vi "Process.vi"(11 "Main Controller":refnum<class "Main Controller Actor.lvclass">) -> ()   [LabVIEW 2021, in "Main Controller Actor.lvclass"]
uses:
  Main Controller Actor.lvclass
  C:/dev/LabVIEW/LabMelee/Source/Re-use Libraries/Minimal Actor Framework/Actors/Base Actor/Actor/Actor.lvclass
  Re-use Libraries/Minimal Actor Framework/Actors/Base Actor/API/Actor API.lvclass
  Main Controller Actor.lvclass/Main Controller Actor.ctl
  View.ctl
  Re-use Libraries/Utility/Utility.lvlib
  Re-use Libraries/Minimal Actor Framework/Actors/Base Actor/Actor/Front Panel State.ctl
  Re-use Libraries/Minimal Actor Framework/Actors/Base Actor/Actor/Actor.lvclass
  Re-use Libraries/Minimal Actor Framework/Messaging/Message/Message.lvclass
  Error Handler/API/Error Handler Actor API.lvclass
  Windows.ctl
  Re-use Libraries/Minimal Actor Framework/Actors/Debugger/Debugger.lvclass
  API/Main Controller Actor API.lvclass
  Views/Main/Main View.lvclass
  Views/Info/Info View.lvclass
  Views/Dev/Dev View.lvclass
  Views/Process Input/Process Input View.lvclass
  Ship.ctl
  Player.ctl
  Player Ship.ctl
panel:
  in  "View":T1
  out "View Title":string
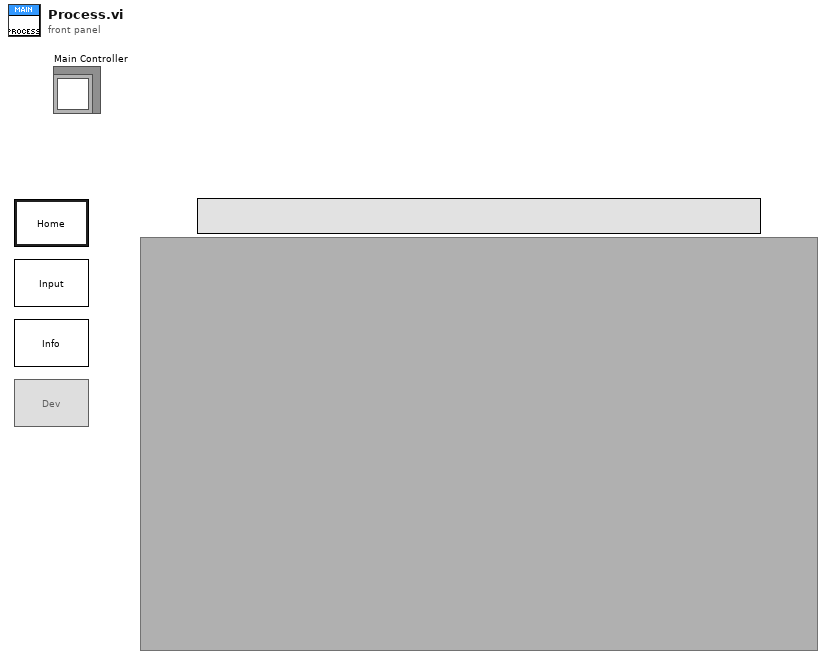
[diagram p1: front panel]
types:
  T1 = typedef "Main Controller Actor.lvclass/View.ctl" = enum32{"Main", "Boolean", "Info", "Dev"}
  T2 = typedef "Actor.lvclass/Front Panel State.ctl" = enum32{"Invalid", "Standard", "Closed", "Hidden", "Minimized", "Maximized"}
  T3 = typedef "Main Controller Actor.lvclass/Player Ship.ctl" = cluster{"Player":T4, "Ship":T5}
  T4 = typedef "Main Controller Actor.lvclass/Player.ctl" = enum16{"1", "2"}
  T5 = typedef "Main Controller Actor.lvclass/Ship.ctl" = enum16{"Arilou", "Chmmr", "Kohrah", "Slylandro"}
  T6 = typedef "Main Controller Actor.lvclass/Windows.ctl" = enum16{"Debugger"}
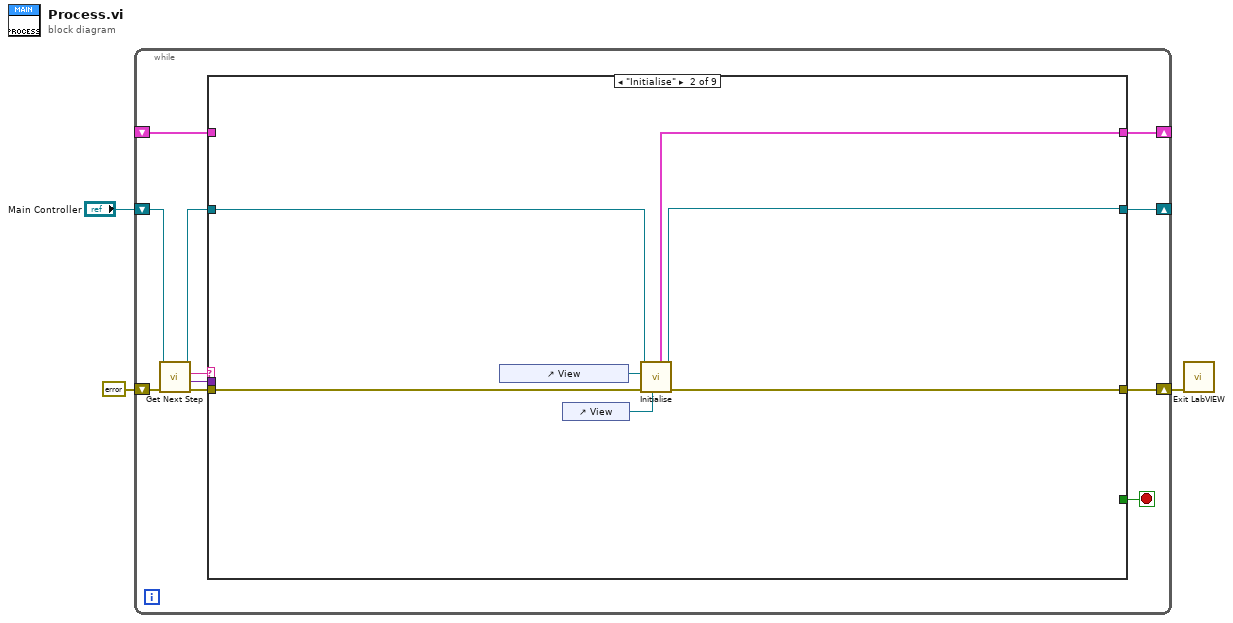
[diagram p0: block diagram]
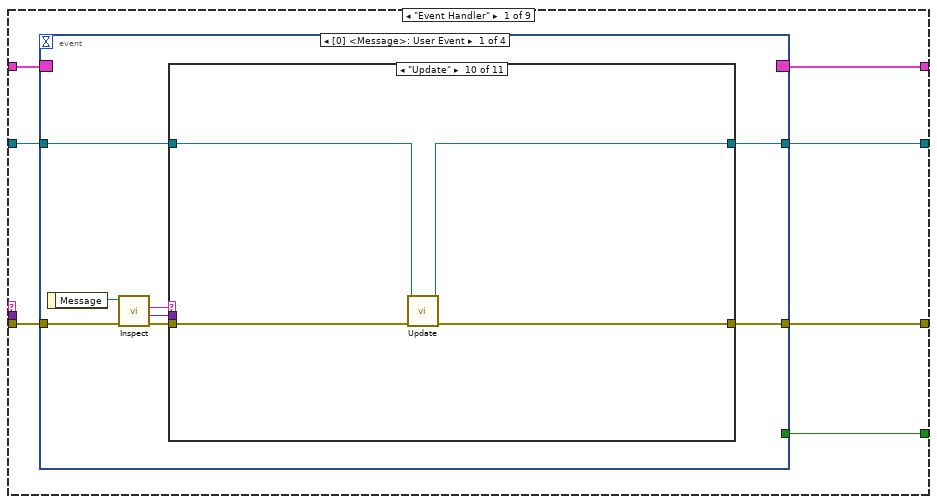
[diagram p2: hidden frame]
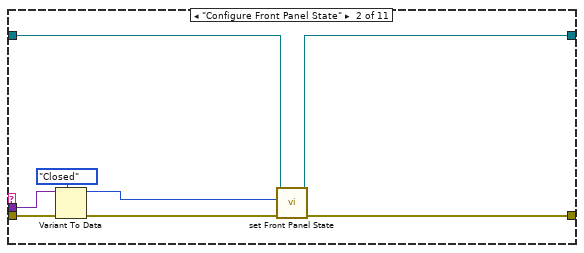
[diagram p4: hidden frame]
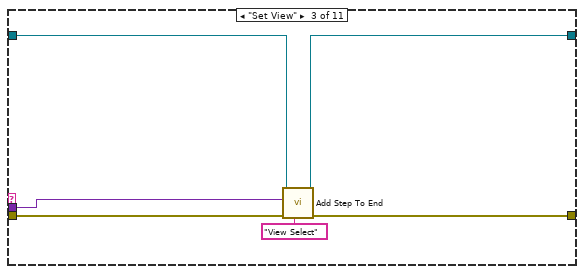
[diagram p5: hidden frame]
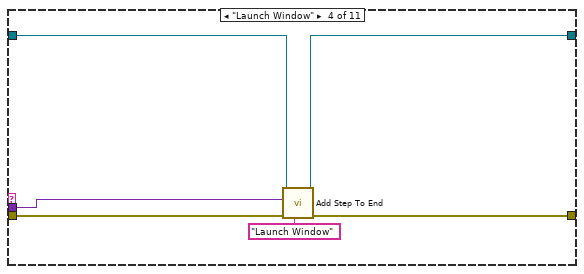
[diagram p6: hidden frame]
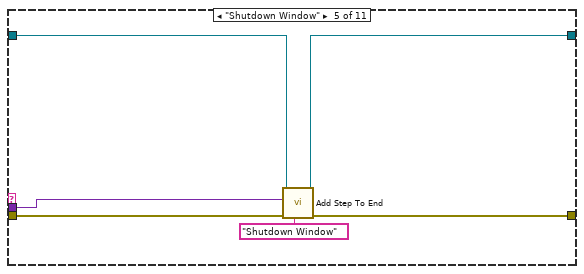
[diagram p7: hidden frame]
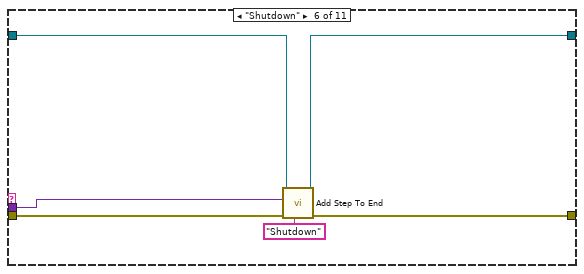
[diagram p8: hidden frame]
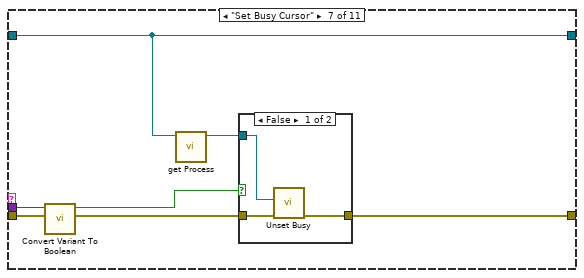
[diagram p9: hidden frame]
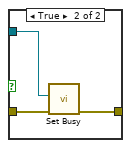
[diagram p10: hidden frame]
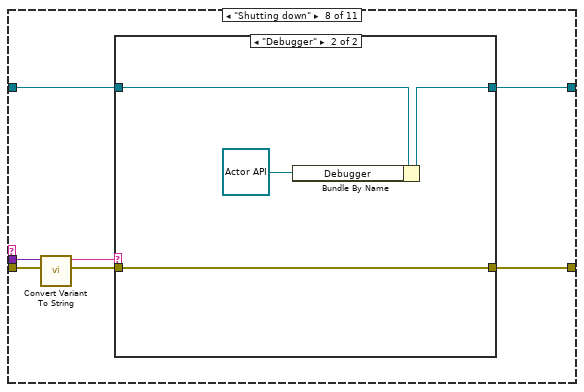
[diagram p11: hidden frame]
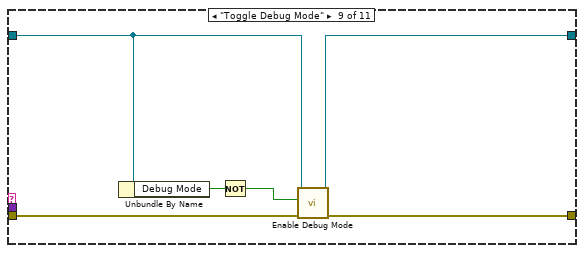
[diagram p13: hidden frame]
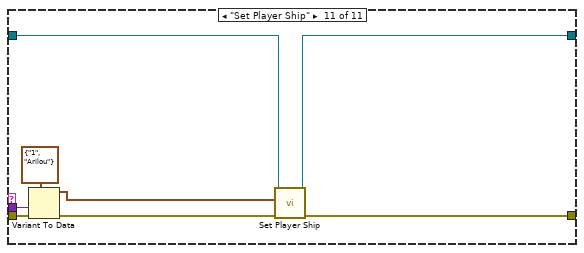
[diagram p14: hidden frame]
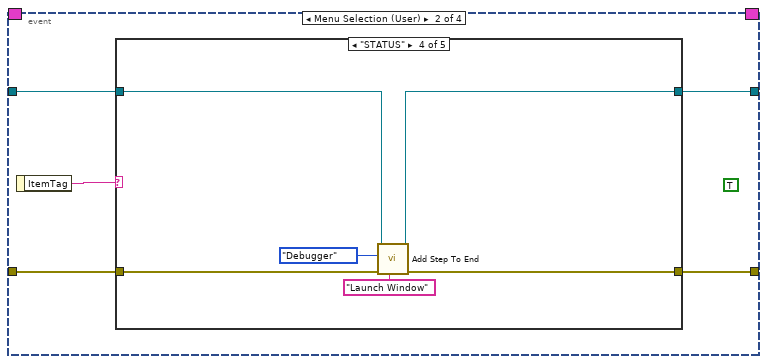
[diagram p15: hidden frame]
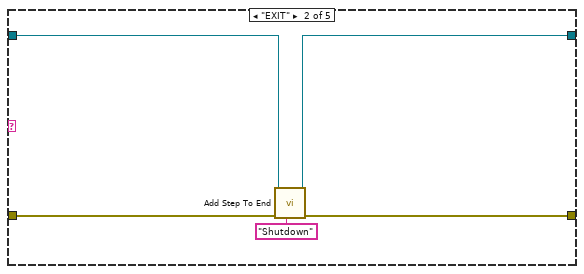
[diagram p17: hidden frame]
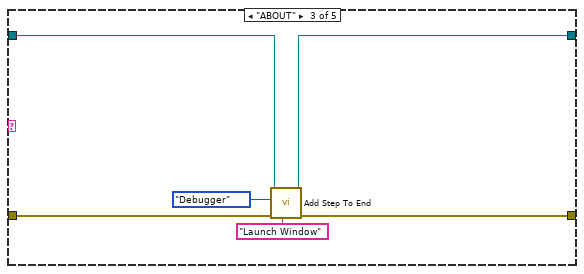
[diagram p18: hidden frame]
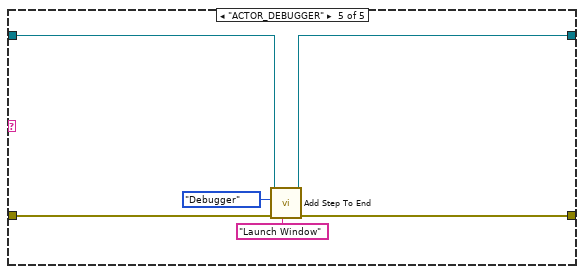
[diagram p19: hidden frame]
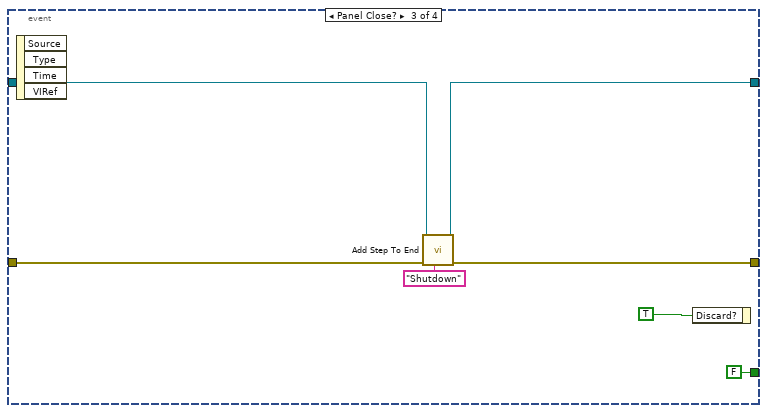
[diagram p20: hidden frame]
diagram:
  n1 = while {
    shift-right: [w9] -> _
    shift-left: "Main Controller" -> [w10]
    shift-right: [w8] -> _
    shift-left: _ -> [w7]
    shift-right: [w5] -> w2
    shift-left: errorcluster {"status"=FALSE, "code"=0, "source"=""} ("error constant") -> [w6]
    stop <- w4 stop-if-true
    n2 = call-dynamic "Get Next Step.vi"("error in (no error)"=w6, "Actor in"=w10) -> ("error out"=w12:errorcluster, "Parameter"=w11:variant, "Step"=w14:string, "Actor out"=w13:refnum<class "Main Controller Actor.lvclass">)  [unwired: 5 in, 1 out]
    n3 = case shown="\"Initialise\"" w14 {
      tunnel: w13 -> [w19 w154 w162 w165 w167 w172 w180 w245 w272]
      tunnel: w12 -> [w18 w152 w159 w164 w168 w170 w182 w242 w275]
      tunnel: w11 -> [_ _ _ _ _ _ w181 w241 w274]
      tunnel: [w20 w149 refnum<class "Main Controller Actor.lvclass"> refnum ("Actor out") w165 w167 w172 w183 w244 w270] -> w9
      tunnel: [w21 w155 w156 w166 w169 w171 w184 w246 w276] -> w8
      tunnel: w7 -> [w15 _ w156 w166 w169 w171 w184 w246 w276]
      tunnel: [w17 w150 w157 w163 w168 w170 w179 w243 w267] -> w5
      tunnel: [w16 _ TRUE _ _ _ _ _ _] -> w4
      frame "Event Handler" {
        n4 = event shown="[0] <Message>: User Event" {
          selector: w15 -> [_ _ _ _]
          dyn-events: [_ _ _ _] -> w21
          timeout: _ -> [_ _ _ _]
          tunnel: [w28 w110 w140 w148] -> w20
          tunnel: w19 -> [w29 w111 w141 w148]
          tunnel: w18 -> [w26 w109 w143 w147]
          tunnel: [w27 w108 w142 w146] -> w17
          tunnel: [_ _ FALSE _] -> w16
          event User Event {
            n5 = event-data() -> ("Message"=w25:refnum<class "Message.lvclass">)  [unwired: 1 in]
            n6 = call "Inspect.vi"("error in (no error)"=w26, "Message in"=w25) -> ("error out"=w24:errorcluster, "Data"=w22:variant, "Name"=w23:string)  [unwired: 5 in, 2 out]
            n7 = case shown="\"Update\"" w23 {
              tunnel: w29 -> [w31 w39 w42 w48 w54 w60 w65 w81 w92 w98 w103]
              tunnel: [w31 w38 w41 w47 w53 w59 w65 w78 w91 w96 w102] -> w28
              tunnel: w24 -> [w30 w35 w45 w51 w57 w63 w70 w83 w95 w99 w106]
              tunnel: [w30 w37 w43 w49 w55 w61 w67 w77 w94 w97 w100] -> w27
              tunnel: w22 -> [_ w36 w40 w46 w52 w58 w69 w82 _ _ w107]
              frame Default {
              }
              frame "Configure Front Panel State" {
                n8 = Variant To Data(error in=w35, type=Front_Panel_State."Closed" ("Front Panel State"), Variant=w36) -> (data=w32:T2, error out=w34:errorcluster)
                n9 = call-dynamic "set Front Panel State.vi"("error in (no error)"=w34, "Front Panel State"=w32, "Actor in"=w39) -> ("error out"=w37:errorcluster, "Actor out"=w38:refnum<class "Main Controller Actor.lvclass">)  [unwired: 7 in]
              }
              frame "Set View" {
                n10 = call-dynamic "Add Step To End.vi"("Step Name"="View Select", "error in (no error)"=w45, "Parameter"=w40, "Actor in"=w42) -> ("error out"=w43:errorcluster, "Actor out"=w41:refnum<class "Main Controller Actor.lvclass">)  [unwired: 6 in]
              }
              frame "Launch Window" {
                n11 = call-dynamic "Add Step To End.vi"("Step Name"="Launch Window", "error in (no error)"=w51, "Parameter"=w46, "Actor in"=w48) -> ("error out"=w49:errorcluster, "Actor out"=w47:refnum<class "Main Controller Actor.lvclass">)  [unwired: 6 in]
              }
              frame "Shutdown Window" {
                n12 = call-dynamic "Add Step To End.vi"("Step Name"="Shutdown Window", "error in (no error)"=w57, "Parameter"=w52, "Actor in"=w54) -> ("error out"=w55:errorcluster, "Actor out"=w53:refnum<class "Main Controller Actor.lvclass">)  [unwired: 6 in]
              }
              frame "Shutdown" {
                n13 = call-dynamic "Add Step To End.vi"("Step Name"="Shutdown", "error in (no error)"=w63, "Parameter"=w58, "Actor in"=w60) -> ("error out"=w61:errorcluster, "Actor out"=w59:refnum<class "Main Controller Actor.lvclass">)  [unwired: 6 in]
              }
              frame "Set Busy Cursor" {
                n14 = call "Convert Variant To Boolean.vi"("error in (no error)"=w70, "Variant"=w69) -> ("error out"=w68:errorcluster, "Boolean"=w66:bool)  [unwired: 8 in]
                n15 = call-dynamic "get Process.vi"("Actor in"=w65) -> ("Process"=w64:refnum<vi>)  [unwired: 9 in, 1 out]
                n16 = case shown="False" w66 {
                  tunnel: w68 -> [w73 w76]
                  tunnel: [w72 w75] -> w67
                  tunnel: w64 -> [w71 w74]
                  frame False {
                    n17 = call <vilib>:"Unset Busy.vi"("error in (no error)"=w73, "VI reference (current VI)"=w71) -> ("error out"=w72:errorcluster)  [unwired: 9 in]
                  }
                  frame True {
                    n18 = call <vilib>:"Set Busy.vi"("error in (no error)"=w76, "VI reference (current VI)"=w74) -> ("error out"=w75:errorcluster)  [unwired: 8 in, 1 out]
                  }
                }
              }
              frame "Shutting down" {
                n19 = call "Convert Variant To String.vi"("error in (no error)"=w83, "Variant"=w82) -> ("error out"=w79:errorcluster, "String"=w80:string)  [unwired: 8 in]
                n20 = case shown="\"Debugger\"" w80 {
                  tunnel: w81 -> [w85 w89]
                  tunnel: w79 -> [w84 w87]
                  tunnel: [w85 w88] -> w78
                  tunnel: [w84 w87] -> w77
                  frame Default {
                  }
                  frame "Debugger" {
                    n21 = Bundle By Name(cluster=w89, "Debugger"=refnum<class "Actor API.lvclass"> refnum ("Windows.About")) -> (w88:refnum<class "Main Controller Actor.lvclass">)
                  }
                }
              }
              frame "Toggle Debug Mode" {
                n22 = Unbundle By Name(w92) -> ("Debug Mode"=w93:bool)
                n23 = Not(x=w93) -> (.not. x?=w90:bool)
                n24 = call "Enable Debug Mode.vi"("error in (no error)"=w95, "Enable Debug"=w90, "Actor in"=w92) -> ("error out"=w94:errorcluster, "Actor out"=w91:refnum<class "Main Controller Actor.lvclass">)  [unwired: 7 in]
              }
              frame "Update" {
                n25 = call "Update.vi"("error in (no error)"=w99, "Main Controller Actor in"=w98) -> ("error out"=w97:errorcluster, "Main Controller Actor out"=w96:refnum<class "Main Controller Actor.lvclass">)  [unwired: 8 in]
              }
              frame "Set Player Ship" {
                n26 = Variant To Data(error in=w106, type=T3 {"Player"=enum."1", "Ship"=enum."Arilou"} ("Cluster"), Variant=w107) -> (data=w104:T3, error out=w101:errorcluster)
                n27 = call "Set Player Ship.vi"("error in (no error)"=w101, "Player Ship"=w104, "Main Controller Actor in"=w103) -> ("error out"=w100:errorcluster, "Main Controller Actor out"=w102:refnum<class "Main Controller Actor.lvclass">)  [unwired: 7 in]
              }
            }
          }
          event Menu Selection (User) {
            (unwired) TRUE
            n28 = event-data() -> ("ItemTag"=w112:string)  [unwired: 1 in]
            n29 = case shown="\"STATUS\"" w112 {
              tunnel: w111 -> [w114 w116 w122 w128 w134]
              tunnel: [w114 w115 w121 w127 w133] -> w110
              tunnel: w109 -> [w113 w118 w124 w130 w136]
              tunnel: [w113 w117 w123 w129 w135] -> w108
              frame Default {
              }
              frame "EXIT" {
                n30 = call-dynamic "Add Step To End.vi"("Step Name"="Shutdown", "error in (no error)"=w118, "Actor in"=w116) -> ("error out"=w117:errorcluster, "Actor out"=w115:refnum<class "Main Controller Actor.lvclass">)  [unwired: 7 in]
              }
              frame "ABOUT" {
                n31 = call-dynamic "Add Step To End.vi"("Step Name"="Launch Window", "error in (no error)"=w124, "Parameter"=Windows."Debugger" ("Windows"), "Actor in"=w122) -> ("error out"=w123:errorcluster, "Actor out"=w121:refnum<class "Main Controller Actor.lvclass">)  [unwired: 6 in]
              }
              frame "STATUS" {
                n32 = call-dynamic "Add Step To End.vi"("Step Name"="Launch Window", "error in (no error)"=w130, "Parameter"=Windows."Debugger" ("Windows"), "Actor in"=w128) -> ("error out"=w129:errorcluster, "Actor out"=w127:refnum<class "Main Controller Actor.lvclass">)  [unwired: 6 in]
              }
              frame "ACTOR_DEBUGGER" {
                n33 = call-dynamic "Add Step To End.vi"("Step Name"="Launch Window", "error in (no error)"=w136, "Parameter"=Windows."Debugger" ("Windows"), "Actor in"=w134) -> ("error out"=w135:errorcluster, "Actor out"=w133:refnum<class "Main Controller Actor.lvclass">)  [unwired: 6 in]
              }
            }
          }
          event Panel Close? {
            n34 = event-data() -> ()  [unwired: 1 in, 4 out]
            n35 = call-dynamic "Add Step To End.vi"("Step Name"="Shutdown", "error in (no error)"=w143, "Actor in"=w141) -> ("error out"=w142:errorcluster, "Actor out"=w140:refnum<class "Main Controller Actor.lvclass">)  [unwired: 7 in]
            n36 = event-data("Discard?"=TRUE) -> ()  [unwired: 1 in, 1 out]
          }
          event Value Change {
            n37 = event-data() -> ()  [unwired: 1 in, 1 out]
            n38 = call "Set View.vi"("error in (no error)"=w147, "View Selection"="View") -> ("error out"=w146:errorcluster)  [unwired: 9 in]
          }
        }
      }
      frame "Initialise" {
        n39 = control-ref of="View"() -> (w151:refnum<vi>)
        n40 = control-ref of="View"() -> (w153:refnum<vi>)
        n41 = call "Initialise.vi"("View"=w153, "error in (no error)"=w152, "View Buttons"=w151, "Main Controller Actor in"=w154) -> ("error out"=w150:errorcluster, "Main Controller Actor out"=w149:refnum<class "Main Controller Actor.lvclass">, "Observers"=w155:cluster{"Actor":refnum<event-registration>})  [unwired: 5 in]
      }
      frame "Shutdown" {
        n42 = Unregister For Events(event registration refnum=w156, error in=w159) -> (error out=w158:errorcluster)
        n43 = call "Final Shutdown.vi"("error in (no error)"=w158, "Main Controller in"=w162) -> ("error out"=w157:errorcluster)  [unwired: 9 in]
      }
      frame "Error Handler" {
        n44 = call "Add LabVIEW Error.vi"("error in (no error)"=w164) -> ("error out"=w163:errorcluster)  [unwired: 10 in]
      }
      frame "Unhandled Step", Default {
      }
      frame "-----------------------" {
        # "Separator"
      }
      frame "View Select" {
        n45 = Unbundle By Name(w180) -> ("Current View"=w178:refnum<class "Actor API.lvclass">, "View State"=w175:T1)
        n46 = Variant To Data(error in=w182, type=View."Main" ("View Selection"), Variant=w181) -> (data=w174:T1, error out=w176:errorcluster)
        n47 = Not Equal?(x=w175, y=w174) -> ()  [unwired: 1 out]
        n48 = case shown="True" TRUE {
          tunnel: [w185 w198] -> w183
          tunnel: w180 -> [w185 w197]
          tunnel: [w186 w196] -> w179
          tunnel: w178 -> [_ w195]
          tunnel: w176 -> [w186 w191]
          tunnel: w174 -> [_ w187]
          frame False {
          }
          frame True {
            n49 = call-dynamic "Shutdown.vi"("error in (no error)"=w191, "Wait For Shutdown (F)"=TRUE, "Actor API in"=w195) -> ("error out"=w194:errorcluster)  [unwired: 8 in]
            n50 = local write "View"(w187) -> ()
            n51 = Bundle By Name(cluster=w197, "View State"=w187) -> (w190:refnum<class "Main Controller Actor.lvclass">)
            n52 = control-ref of="View"() -> (w192:refnum<vi>)
            n53 = case shown="\"Dev\"" w187 {
              selector: w187 -> [w200 _ _ _ _]
              tunnel: [w203 w206 w221 w229 w237] -> w196
              tunnel: w192 -> [_ w213 w220 w228 w236]
              tunnel: 10000 ("Launch Timeout [ms]") -> [_ w212 w219 w227 w235]
              tunnel: w194 -> [w204 w211 w218 w226 w234]
              tunnel: w190 -> [w205 w208 w214 w222 w233]
              tunnel: [w205 w207 w217 w225 w232] -> w198
              tunnel: [_ w209 w215 w223 w230] -> w188
              frame Default {
                n54 = Format Into String(format string="Cannot start SubPanel Actor %s", w200) -> (resulting string=w199:string)  [unwired: 2 in, 1 out]
                n55 = call <vilib>:"Error Cluster From Error Code.vi"("error in (no error)"=w204, "error message (\"\")"=w199, "error code (0)"=42) -> ("error out"=w203:errorcluster)  [unwired: 6 in]
              }
              frame "Main" {
                n56 = call "Launch.vi"("Sub Panel"=w213, "Launch Timeout [ms]"=w212, "error in (no error)"=w211) -> ("error out"=w206:errorcluster, "Title"=w209:string, "Actor API out"=w210:refnum<class "Actor API.lvclass">)  [unwired: 5 in, 1 out]
                n57 = Bundle By Name(cluster=w208, "Current View"=w210) -> (w207:refnum<class "Main Controller Actor.lvclass">)
              }
              frame "Boolean" {
                n58 = call "Launch.vi"("Sub Panel"=w220, "Launch Timeout [ms]"=w219, "error in (no error)"=w218) -> ("error out"=w221:errorcluster, "Title"=w215:string, "Actor API out"=w216:refnum<class "Actor API.lvclass">)  [unwired: 5 in, 1 out]
                n59 = Bundle By Name(cluster=w214, "Current View"=w216) -> (w217:refnum<class "Main Controller Actor.lvclass">)
              }
              frame "Info" {
                n60 = call "Launch.vi"("Sub Panel"=w228, "Launch Timeout [ms]"=w227, "error in (no error)"=w226) -> ("error out"=w229:errorcluster, "Title"=w223:string, "Actor API out"=w224:refnum<class "Actor API.lvclass">)  [unwired: 5 in, 1 out]
                n61 = Bundle By Name(cluster=w222, "Current View"=w224) -> (w225:refnum<class "Main Controller Actor.lvclass">)
              }
              frame "Dev" {
                n62 = call "Launch.vi"("Sub Panel"=w236, "Launch Timeout [ms]"=w235, "error in (no error)"=w234) -> ("error out"=w237:errorcluster, "Title"=w230:string, "Actor API out"=w231:refnum<class "Actor API.lvclass">)  [unwired: 5 in, 1 out]
                n63 = Bundle By Name(cluster=w233, "Current View"=w231) -> (w232:refnum<class "Main Controller Actor.lvclass">)
              }
            }
            "View Title" <- w188
          }
        }
      }
      frame "Launch Window" {
        # "This is use to launch windows that are not tied to a specific view"
        n64 = Variant To Data(error in=w242, type=Windows."Debugger" ("Windows"), Variant=w241) -> (data=w238:T6, error out=w239:errorcluster)
        n65 = case shown="\"Debugger\"" w238 {
          tunnel: w239 -> [w247 w254]
          tunnel: w245 -> [w248 w252]
          tunnel: [w248 w251] -> w244
          tunnel: [w247 w249] -> w243
          frame Default {
          }
          frame "Debugger" {
            n66 = Unbundle By Name(w252) -> ("Debugger"=w250:refnum<class "Actor API.lvclass">)
            n67 = call-dynamic "Check If Valid.vi"("Actor API in"=w250) -> ("Valid"=w253:bool)  [unwired: 10 in]
            n68 = case shown="False" w253 {
              tunnel: w254 -> [w259 w264]
              tunnel: w252 -> [w256 w263]
              tunnel: [w260 w263] -> w251
              tunnel: w250 -> [_ w265]
              tunnel: [w257 w261] -> w249
              frame False {
                n69 = call "get Request Channel.vi"("Actor in"=w256) -> ("Request Channel"=w255:refnum<class "Messenger.lvclass">)  [unwired: 8 in, 2 out]
                n70 = call "Launch.vi"("error in (no error)"=w259, "Response Channel"=w255) -> ("error out"=w257:errorcluster, "Actor API out"=w258:refnum<class "Actor API.lvclass">)  [unwired: 8 in]
                n71 = Bundle By Name(cluster=w256, "Debugger"=w258) -> (w260:refnum<class "Main Controller Actor.lvclass">)
              }
              frame True {
                n72 = call-dynamic "Configure Front Panel State.vi"("error in (no error)"=w264, "Front Panel State"=Front_Panel_State."Standard", "Actor API in"=w265) -> ("error out"=w261:errorcluster)  [unwired: 8 in]
              }
            }
          }
        }
      }
      frame "Shutdown Window" {
        n73 = Variant To Data(error in=w275, type=Windows."Debugger" ("Windows"), Variant=w274) -> (data=w271:T6, error out=w268:errorcluster)
        n74 = case shown="\"Debugger\"" w271 {
          tunnel: w272 -> [w284]
          tunnel: [w282] -> w270
          tunnel: [w281] -> w266
          frame "Debugger" {
            n75 = Unbundle By Name(w284) -> ("Debugger"=w281:refnum<class "Actor API.lvclass">)
            n76 = Bundle By Name(cluster=w284, "Debugger"=refnum<class "Actor API.lvclass"> refnum ("Windows.Status")) -> (w282:refnum<class "Main Controller Actor.lvclass">)
          }
        }
        n77 = call-dynamic "Check If Valid.vi"("Actor API in"=w266) -> ("Valid"=w269:bool)  [unwired: 10 in]
        n78 = case shown="True" w269 {
          tunnel: w268 -> [w277 w280]
          tunnel: [w277 w279] -> w267
          tunnel: w266 -> [_ w278]
          frame False {
          }
          frame True {
            n79 = call-dynamic "Shutdown.vi"("error in (no error)"=w280, "Actor API in"=w278) -> ("error out"=w279:errorcluster)  [unwired: 9 in]
          }
        }
      }
    }
  }
  n80 = call "Exit LabVIEW.vi"("Data Flow Dependency"=w2) -> ()  [unwired: 11 in]
